vi "InitLog.vi"(8 "error control":errorcluster, 9 "Unit":string[](array[string]), 10 "Property":string[](array[string]), 11 "file path (use dialog)":path) -> (0 "error indicator":errorcluster, 3 "refnum out":refnum<file>)   [LabVIEW 2014]
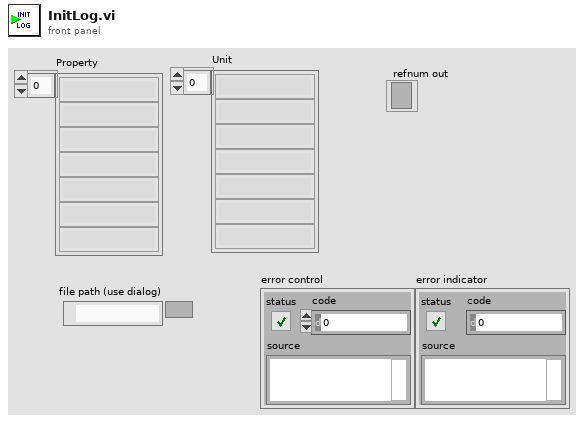
[diagram p1: front panel]
types:
  T1 = enum16{"open", "replace", "create", "open or create", "replace or create", "replace or create with confirmation"}
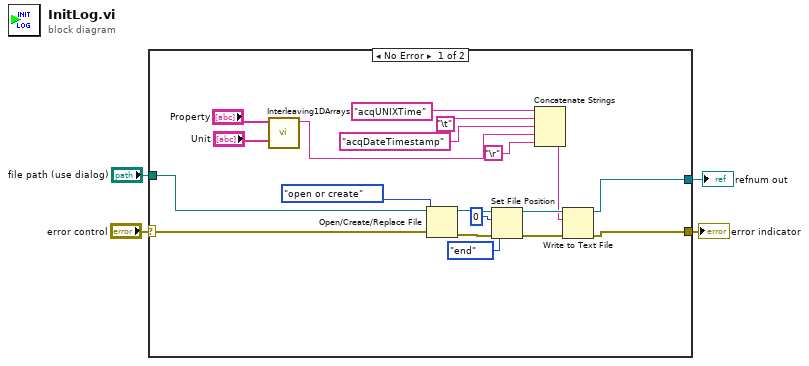
[diagram p0: block diagram]
diagram:
  n1 = case shown="No Error" "error control" {
    selector: "error control" -> [w10 w24]
    tunnel: [w12 w24] -> w3
    tunnel: [w11 _] -> w2
    tunnel: "file path (use dialog)" -> [w9 _]
    frame No Error {
      n2 = call "Interleaving1DArrays.vi"("Unit"="Unit", "Property"="Property") -> ("Column Header"=w7:string)  [unwired: 9 in]
      n3 = Open/Create/Replace File(file path (use dialog)=w9, error in=w10, operation (0:open)=T1."open or create") -> (refnum out=w21:refnum<file>, error out=w18:errorcluster)  [unwired: 3 in, 1 out]
      n4 = Set File Position(offset (in bytes) (0)=i64 0, refnum=w21, from (0:start)=enum16{"start", "end", "current"}."end", error in=w18) -> (refnum out=w20:refnum<file>, error out=w19:errorcluster)
      n5 = Concatenate Strings("acqUNIXTime" ("string"), "\t", "acqDateTimestamp" ("string"), w7, "\r") -> (w8:string)
      n6 = Write to Text File(file (use dialog)=w20, text=w8, error in=w19) -> (refnum out=w11:refnum<file>, error out=w12:errorcluster)  [unwired: 1 in, 1 out]
    }
    frame Error {
    }
  }
  "error indicator" <- w3
  "refnum out" <- w2
